vi "CloseLEDStrip.vi"(8 "error in (no error)":errorcluster, 11 "LEDStripRef in":T1={"PWM Rate (Hz)"=1000.0, "Max Duty Cycle"=0.0, "DigitalOutputRed"={"Digital Module"=enum."Digital Module 1", "DIO Channel"=enum."DIO 1", "DevStatus"={"status"=FALSE, "code"=0, "source"=""}}, "DigitalOutputGreen"={"Digital Module"=enum."Digital Module 1", "DIO Channel"=enum."DIO 1", "DevStatus"={"status"=FALSE, "code"=0, "source"=""}}, "DigitalOutputBlue"={"Digital Module"=enum."Digital Module 1", "DIO Channel"=enum."DIO 1", "DevStatus"={"status"=FALSE, "code"=0, "source"=""}}, "DevStatus"={"status"=FALSE, "code"=0, "source"=""}}) -> (0 "error out":errorcluster)   [LabVIEW 2013]
uses:
  LEDStripRef.ctl
  <vilib>/Rock Robotics/WPI/DigitalOutput/WPI_DigitalOutputDevRef.ctl
  <vilib>/Rock Robotics/SystemInterfaces/Typedef/FPGA_TypedefDigitalModule.ctl
  <vilib>/Rock Robotics/SystemInterfaces/DIO/FPGA_DIOChannel.ctl
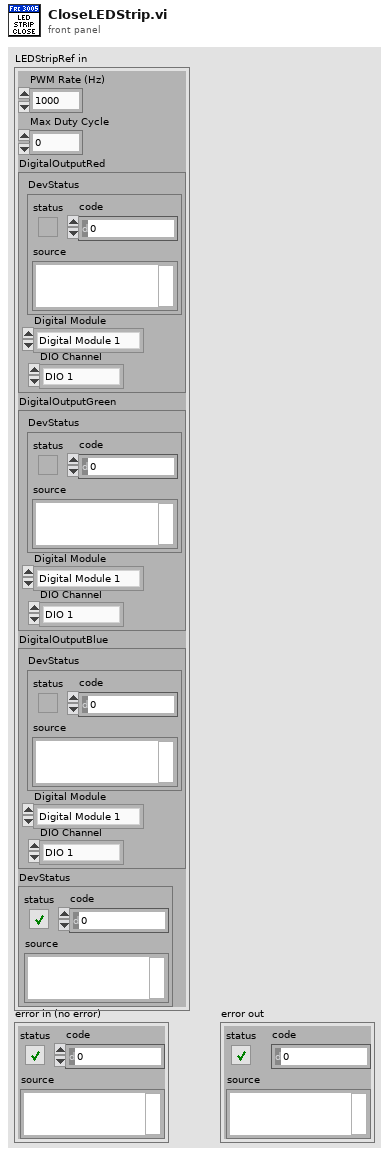
[diagram p1: front panel]
types:
  T1 = typedef "LEDStripRef.ctl" = cluster{"PWM Rate (Hz)":sgl, "Max Duty Cycle":sgl, "DigitalOutputRed":T2, "DigitalOutputGreen":T2, "DigitalOutputBlue":T2, "DevStatus":errorcluster}
  T2 = typedef "WPI_DigitalOutputDevRef.ctl" = cluster{"Digital Module":T3, "DIO Channel":T4, "DevStatus":errorcluster}
  T3 = typedef "FPGA_TypedefDigitalModule.ctl" = enum16{"Digital Module 1", "Digital Module 2"}
  T4 = typedef "FPGA_DIOChannel.ctl" = enum8{"DIO 1", "DIO 2", "DIO 3", "DIO 4", "DIO 5", "DIO 6", "DIO 7", "DIO 8", "DIO 9", "DIO 10", "DIO 11", "DIO 12", "DIO 13", "DIO 14", "Invalid"}
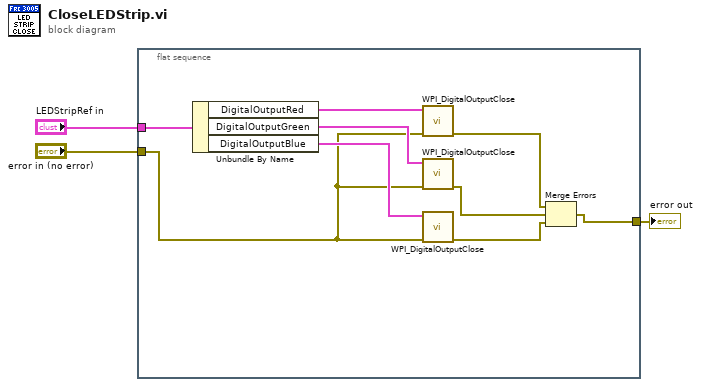
[diagram p0: block diagram]
diagram:
  n1 = flat-sequence {
    tunnel: "LEDStripRef in" -> [w12]
    tunnel: "error in (no error)" -> [w8]
    tunnel: [w4] -> w3
    frame #0 {
      n2 = Unbundle By Name(w12) -> ("DigitalOutputRed"=w11:T2, "DigitalOutputGreen"=w10:T2, "DigitalOutputBlue"=w9:T2)
      n3 = call <vilib>:"WPI_DigitalOutputClose.vi"("error in (no error)"=w8, "DigitalOutputDevRef"=w11) -> ("error out"=w7:errorcluster)  [unwired: 9 in]
      n4 = call <vilib>:"WPI_DigitalOutputClose.vi"("error in (no error)"=w8, "DigitalOutputDevRef"=w10) -> ("error out"=w6:errorcluster)  [unwired: 9 in]
      n5 = call <vilib>:"WPI_DigitalOutputClose.vi"("error in (no error)"=w8, "DigitalOutputDevRef"=w9) -> ("error out"=w5:errorcluster)  [unwired: 9 in]
      n6 = Merge Errors(w7, w6, w5) -> (w4:errorcluster)
    }
  }
  "error out" <- w3
